vi "Untitled 5.vi"() -> ()   [LabVIEW 2017]
panel:
  out "Array":dbl[](array[numeric])
  out "Array 3":dbl[](array[numeric])
  out "Array 2":dbl[][](array[numeric])
  out "1D Array":dbl[](array[numeric])
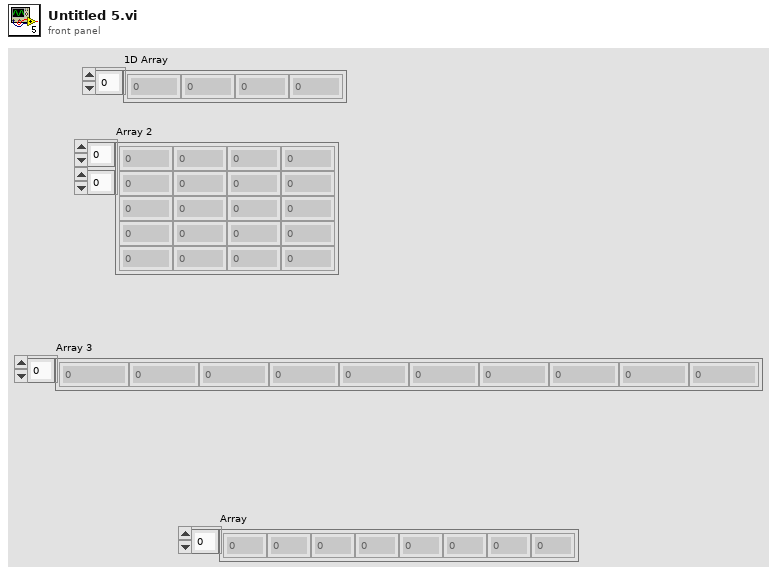
[diagram p1: front panel]
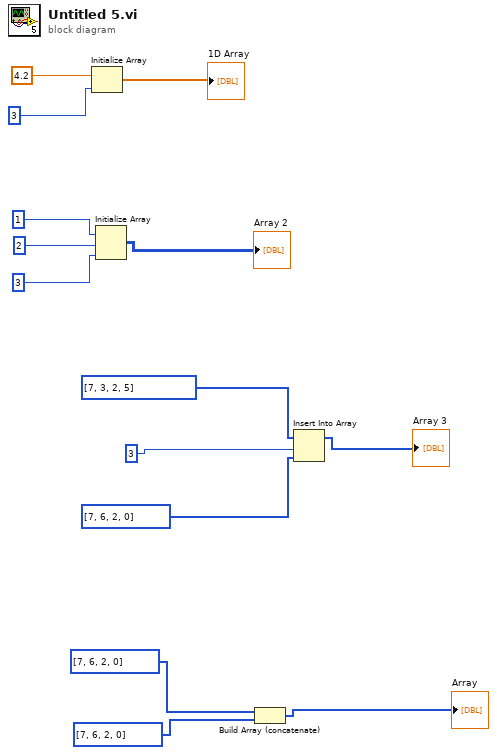
[diagram p0: block diagram]
diagram:
  n1 = Initialize Array(4.2, 3) -> (→"1D Array":dbl[])
  n2 = Initialize Array(1, 2, 3) -> (→"Array 2":i32[][])
  n3 = Build Array (concatenate)(i32[] [7, 6, 2, 0], i32[] [7, 6, 2, 0]) -> (→"Array":i32[])
  n4 = Insert Into Array(array=i32[] [7, 3, 2, 5], index=3, new element=i32[] [7, 6, 2, 0]) -> (→"Array 3":i32[])
